vi "write_loaded_vars_to_controls.vi"(7 "Variable Values":T1, 11 "error in (no error)":errorcluster, 13 "Variable References":T2) -> (8 "Variable Values Out":T1, 15 "error out":errorcluster)   [LabVIEW 2023]
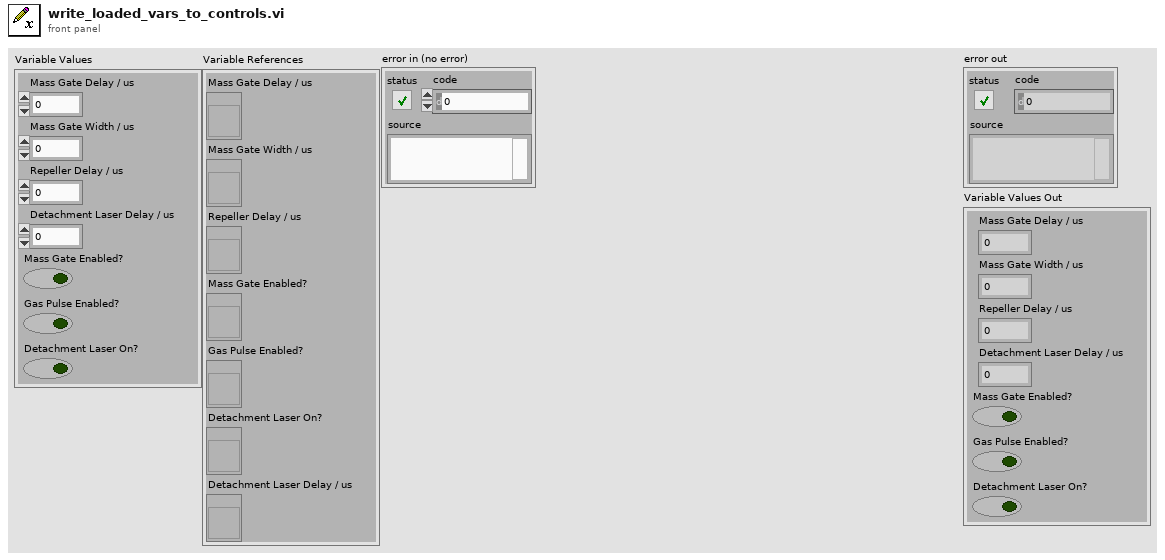
[diagram p1: front panel]
types:
  T1 = cluster{"Mass Gate Delay / us":dbl, "Mass Gate Width / us":dbl, "Repeller Delay / us":dbl, "Detachment Laser Delay / us":dbl, "Mass Gate Enabled?":bool, "Gas Pulse Enabled?":bool, "Detachment Laser On?":bool}
  T2 = cluster{"Mass Gate Delay / us":refnum<vi>, "Mass Gate Width / us":refnum<vi>, "Repeller Delay / us":refnum<vi>, "Mass Gate Enabled?":refnum<vi>, "Gas Pulse Enabled?":refnum<vi>, "Detachment Laser On?":refnum<vi>, "Detachment Laser Delay / us":refnum<vi>}
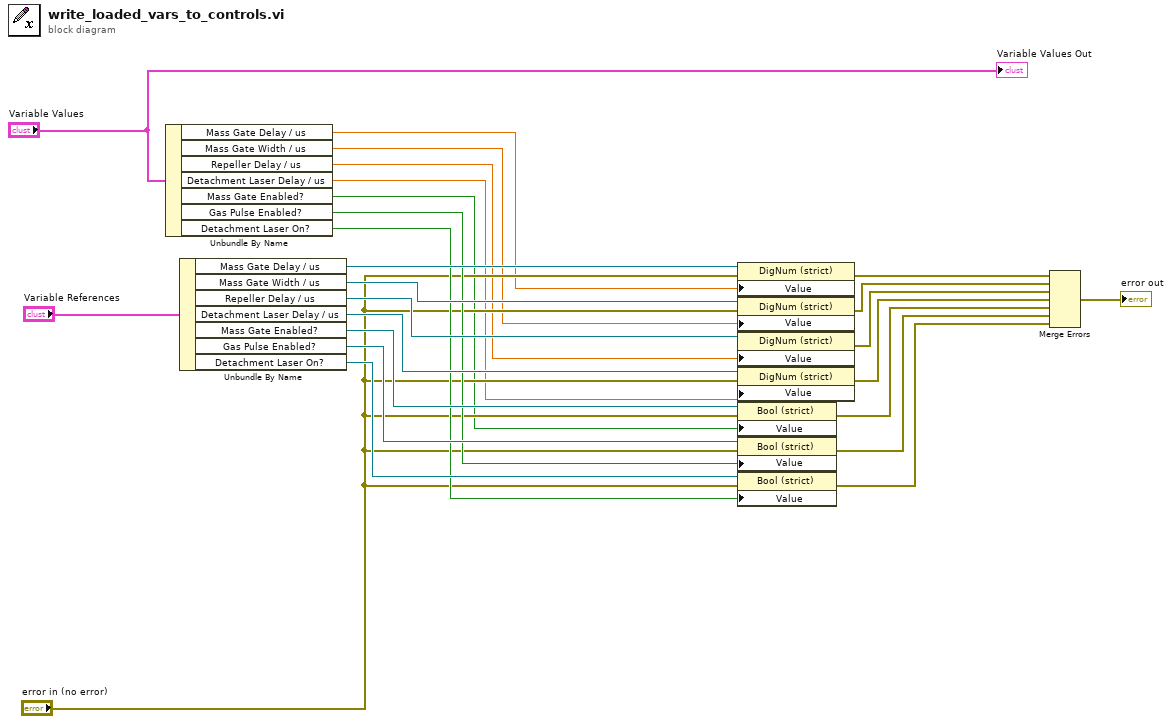
[diagram p0: block diagram]
diagram:
  n1 = Unbundle By Name("Variable Values") -> ("Mass Gate Delay / us"=w9:dbl, "Mass Gate Width / us"=w10:dbl, "Repeller Delay / us"=w11:dbl, "Detachment Laser Delay / us"=w12:dbl, "Mass Gate Enabled?"=w13:bool, "Gas Pulse Enabled?"=w15:bool, "Detachment Laser On?"=w16:bool)
  n2 = Unbundle By Name("Variable References") -> ("Mass Gate Delay / us"=w24:refnum<vi>, "Mass Gate Width / us"=w23:refnum<vi>, "Repeller Delay / us"=w22:refnum<vi>, "Detachment Laser Delay / us"=w21:refnum<vi>, "Mass Gate Enabled?"=w20:refnum<vi>, "Gas Pulse Enabled?"=w19:refnum<vi>, "Detachment Laser On?"=w18:refnum<vi>)
  n3 = property class="DigNum (strict)"(reference=w24, error in="error in (no error)", "Value"=w9) -> (error out=w8:errorcluster)  [unwired: 1 out]
  n4 = property class="DigNum (strict)"(reference=w23, error in="error in (no error)", "Value"=w10) -> (error out=w7:errorcluster)  [unwired: 1 out]
  n5 = property class="DigNum (strict)"(reference=w22, "Value"=w11) -> (error out=w6:errorcluster)  [unwired: 1 in, 1 out]
  n6 = property class="DigNum (strict)"(reference=w21, error in="error in (no error)", "Value"=w12) -> (error out=w5:errorcluster)  [unwired: 1 out]
  n7 = property class="Bool (strict)"(reference=w20, error in="error in (no error)", "Value"=w13) -> (error out=w4:errorcluster)  [unwired: 1 out]
  n8 = property class="Bool (strict)"(reference=w19, error in="error in (no error)", "Value"=w15) -> (error out=w3:errorcluster)  [unwired: 1 out]
  n9 = property class="Bool (strict)"(reference=w18, error in="error in (no error)", "Value"=w16) -> (error out=w2:errorcluster)  [unwired: 1 out]
  n10 = Merge Errors(w8, w7, w6, w5, w4, w3, w2) -> (→"error out":errorcluster)
  "Variable Values Out" <- "Variable Values"
